vi "Start Streaming.vi"(8 "error in (no error)":errorcluster, 9 "Camera Settings":T1={"Exposure Time (ms)"=100.0, "Binning"=enum."2x2", "Scan Mode"=-1, "Frames to Acquire"=1000.0, "Pixel Correction"=FALSE, "Frames to Skip"=1, "File Path"=path "", "Duty cycle"=1.0, "ALEX"=FALSE, "Shutter Enable"=[], "fluidics trigger frame"=0, "Bit Depth"=16, "Image Width (px)"=0, "Image Height (px)"=0, "Horizontal Offset (px)"=0, "Vertical Offset (px)"=0} {"fluidics trigger frame" max=60000 step=1; "Exposure Time (ms)" min=1.0 max=10000.0 step=1.0}, 11 "Synchronization Device in":refnum<class "Sync Device.lvclass">) -> (0 "error out":errorcluster, 3 "Synchronization Device out":refnum<class "Sync Device.lvclass">)   [LabVIEW 2023, in "Sync Device.lvlib" / "Sync Device.lvclass"]
uses:
  Sync Device.lvclass
  Resources/Type Defs/Camera Settings.ctl
  Sync Device.lvclass/Sync Device.ctl
  <vilib>/ActorFramework/Actor/Actor.lvclass
  <vilib>/Utility/error.llb/DialogType.ctl
  Application Messages/Record Button Off Msg/Cancel Operation Msg.lvclass
  C:/FlashGordon/Development/Hardware/Device/Device.lvclass
  C:/Program Files/National Instruments/LabVIEW 2023/vi.lib/ActorFramework/Actor/Actor.lvclass
  C:/FlashGordon/Development/Hardware/Sync Device/Sync Device.lvclass
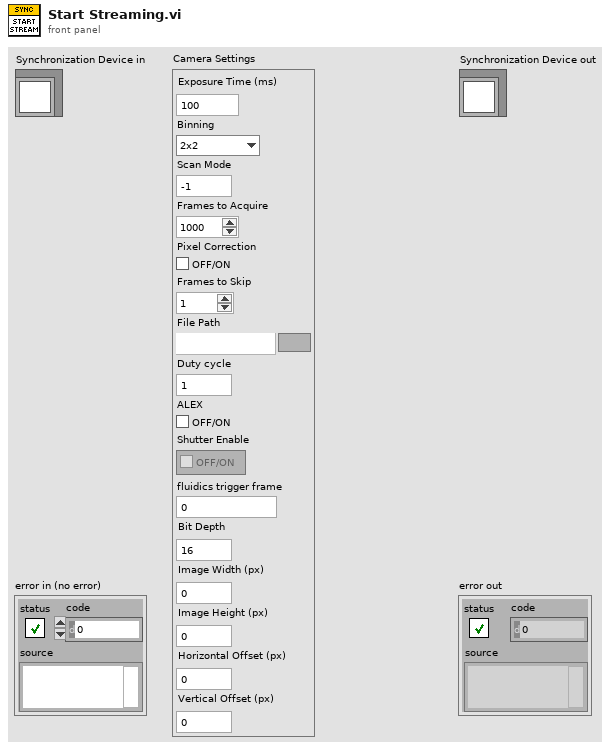
[diagram p1: front panel]
types:
  T1 = typedef "Camera Settings.ctl" = cluster{"Exposure Time (ms)":dbl, "Binning":enum16{"1x1", "2x2", "4x4"}, "Scan Mode":i32, "Frames to Acquire":dbl, "Pixel Correction":bool, "Frames to Skip":u32, "File Path":path, "Duty cycle":dbl, "ALEX":bool, "Shutter Enable":bool[], "fluidics trigger frame":u16, "Bit Depth":u16, "Image Width (px)":u16, "Image Height (px)":u16, "Horizontal Offset (px)":u16, "Vertical Offset (px)":u16}
  T2 = typedef "DialogType.ctl" = u16
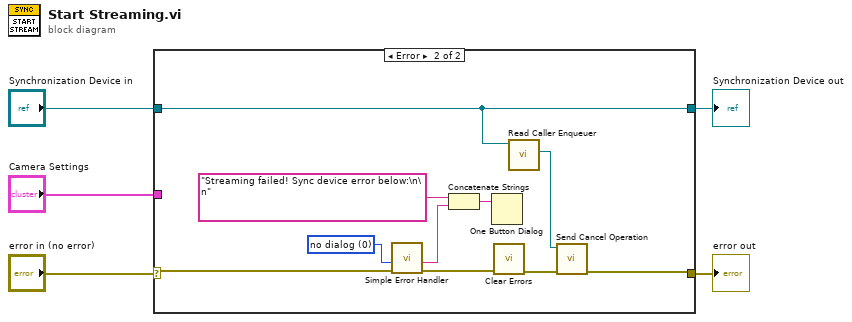
[diagram p0: block diagram]
diagram:
  n1 = case shown="Error" "error in (no error)" {
    selector: "error in (no error)" -> [w6 w14]
    tunnel: [w6 w9] -> w4
    tunnel: [w7 w10] -> w2
    tunnel: "Synchronization Device in" -> [w7 w10]
    tunnel: "Camera Settings" -> [_ _]
    frame No Error {
    }
    frame Error {
      w13 = T2 0 items=["no dialog", "OK message", "continue or stop message", "OK message + warnings", "continue/stop + warnings"] ("type of dialog (OK msg:1)")
      n2 = call <vilib>:"Simple Error Handler.vi"("type of dialog (OK msg:1)"=w13, "error in (no error)"=w14) -> ("source out"=w8:string, "error out"=w12:errorcluster)  [unwired: 3 in, 3 out]
      n3 = Concatenate Strings("Streaming failed! Sync device error below:\n\n" ("string"), w8) -> (w17:string)
      n4 = One Button Dialog(message=w17) -> ()  [unwired: 1 in, 1 out]
      n5 = call <vilib>:"Clear Errors.vi"("error in (no error)"=w12) -> ("error out"=w11:errorcluster)  [unwired: 5 in, 1 out]
      n6 = call <vilib>:"Read Caller Enqueuer.vi"("Actor"=w10) -> ("Caller Enqueuer"=w15:refnum<class "Message Enqueuer.lvclass">)  [unwired: 10 in]
      n7 = call "Send Cancel Operation.vi"("error in (no error)"=w11, "Message Enqueuer"=w15) -> ("error out"=w9:errorcluster)  [unwired: 8 in, 1 out]
    }
  }
  "error out" <- w4
  "Synchronization Device out" <- w2
